vi "EIP IO Folder.vi"(8 "error in (no error)":errorcluster, 11 "Node Ptr":T1 format="%.0x") -> (0 "error out":errorcluster)   [LabVIEW 2011, in "Ethernet IP Custom Device Custom Device.lvlib"]
uses:
  Ethernet IP Custom Device Custom Device.lvlib
  <vilib>/NI Veristand/Custom Device API/Custom Device Item Ref.ctl
  <vilib>/NI Veristand/Custom Device API/Custom Device Channel.ctl
  <vilib>/NI Veristand/Custom Device API/Custom Device Channel Type.ctl
  Ethernet IP Global Strings.vi
  <vilib>/NI Veristand/Custom Device API/Get Item Property (Boolean).vi
  Ethernet IP Global GUIDs.vi
  <vilib>/NI Veristand/Custom Device API/Custom Device API.lvlib
panel:
  in  "Add Channel":bool
  in  "Header":cluster{"Section Name":string}={"Section Name"="Custom Device Item Settings"}
  out "Description":string
  out "Name":string
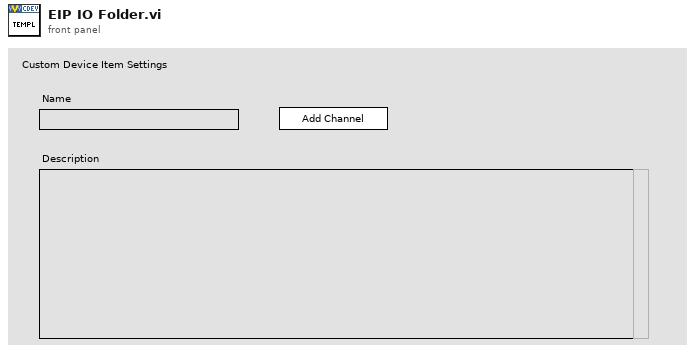
[diagram p1: front panel]
types:
  T1 = typedef "Custom Device API.lvlib/Custom Device Item Ref.ctl" = u64
  T2 = typedef "Custom Device API.lvlib/Custom Device Item Info.ctl" = cluster{"Name":string, "Is Channel":bool, "GUID":string}
  T3 = typedef "Custom Device API.lvlib/Custom Device Channel.ctl" = cluster{"Type":T4, "Units":string, "Default Value":dbl, "Faultable":bool, "Scalable":bool}
  T4 = typedef "Custom Device API.lvlib/Custom Device Channel Type.ctl" = enum16{"Input", "Output"}
  T5 = typedef "Custom Device API.lvlib/Custom Device Commands.ctl" = enum16{"Default", "Item renamed", "Shutdown", "Dynamic button pressed"}
  T6 = typedef "Ethernet IP Custom Device Custom Device.lvlib/L5K Data Types.ctl" = enum16{"SINT", "INT", "DINT", "REAL", "BOOL"}
  T7 = cluster{"Channel Name":string, "Tag Name":string, "Number of Elements":u16, "Data Type":T6}
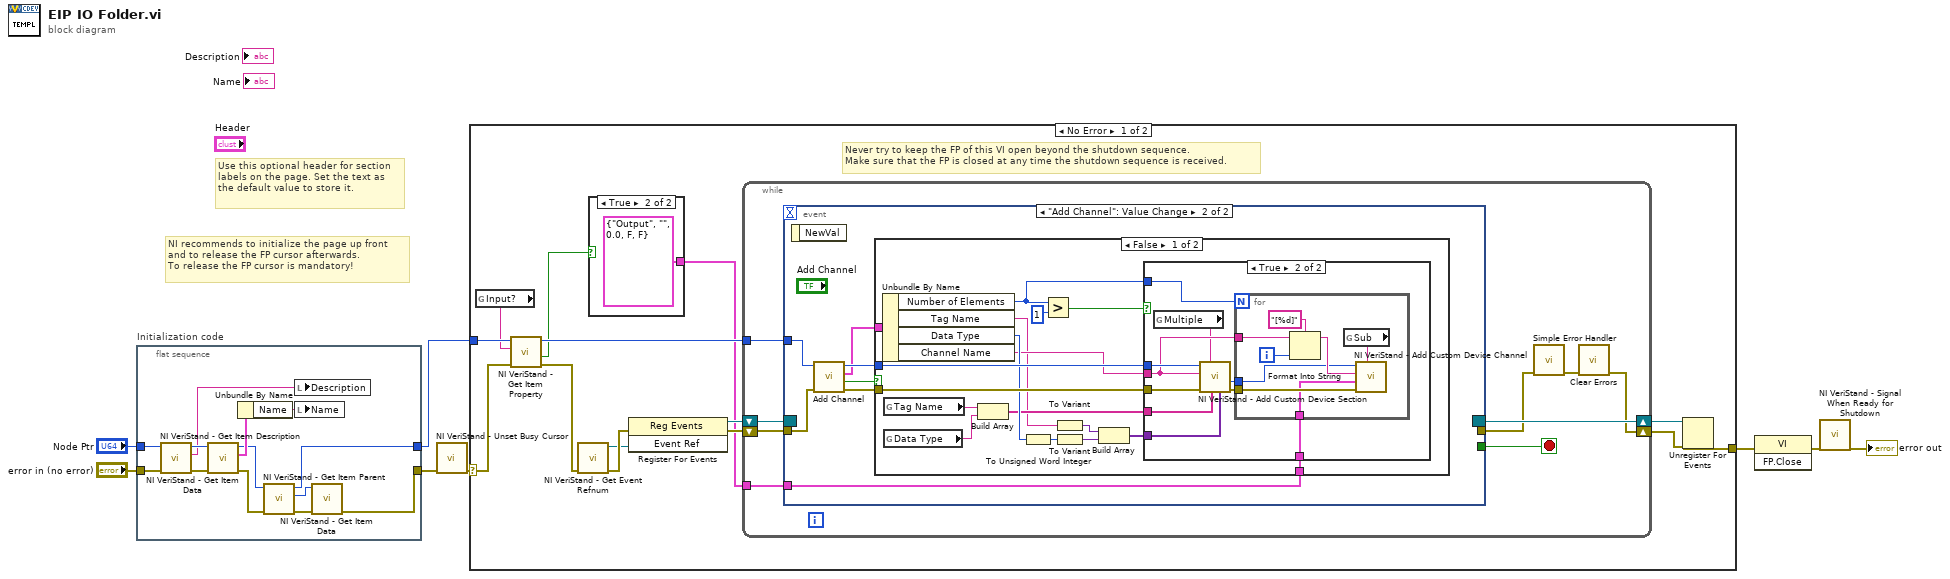
[diagram p0: block diagram]
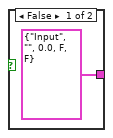
[diagram p2: hidden frame]
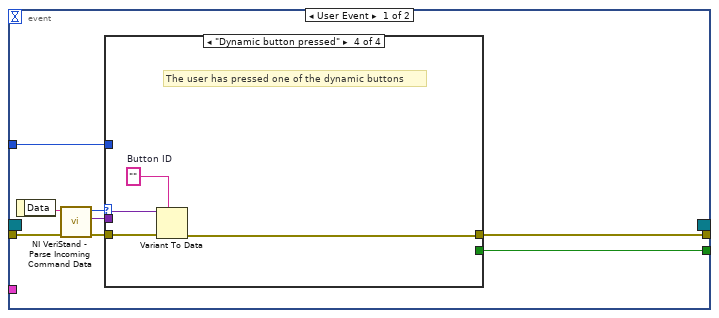
[diagram p3: hidden frame]
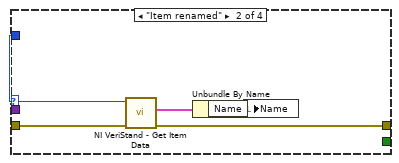
[diagram p5: hidden frame]
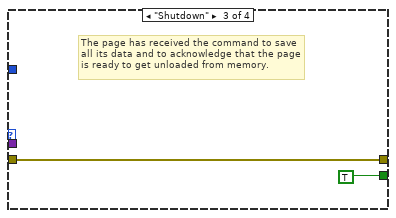
[diagram p6: hidden frame]
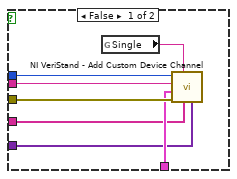
[diagram p7: hidden frame]
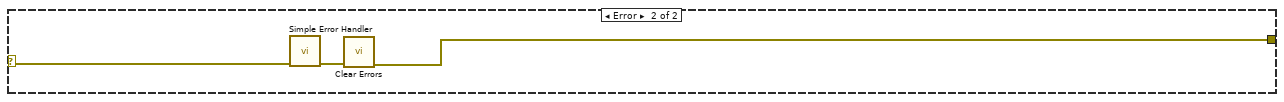
[diagram p9: hidden frame]
diagram:
  # "Use this optional header for section labels on the page. Set the text as the default value to store it."
  # "NI recommends to initialize the page up front\nand to release the FP cursor afterwards.\nTo release the FP cursor is mandatory!"
  n1 = flat-sequence "Initialization code" {
    tunnel: "error in (no error)" -> [w20]
    tunnel: "Node Ptr" -> [w19]
    tunnel: [w12] -> w2
    tunnel: [w10] -> w1
    frame #0 {
      n2 = call <vilib>:"NI VeriStand - Get Item Description.vi"("error in (no error)"=w20, "Item Ref in"=w19) -> ("error out"=w17:errorcluster, "Description"=w18:string, "Item Ref out"=w21:T1)  [unwired: 7 out]
      n3 = call <vilib>:"NI VeriStand - Get Item Data.vi"("error in (no error)"=w17, "Item Ref in"=w21) -> ("error out"=w14:errorcluster, "Item Info"=w16:T2, "Item Ref out"=w13:T1)  [unwired: 7 out]
      n4 = Unbundle By Name(w16) -> ("Name"=w15:string)
      n5 = call <vilib>:"NI VeriStand - Get Item Parent.vi"("error in (no error)"=w14, "Item Ref in"=w13) -> ("error out"=w11:errorcluster, "Parent Ref"=w9:T1, "Item Ref out"=w12:T1)  [unwired: 6 in, 1 out]
      n6 = local write "Description"(w18) -> ()
      n7 = local write "Name"(w15) -> ()
      n8 = call <vilib>:"NI VeriStand - Get Item Data.vi"("error in (no error)"=w11, "Item Ref in"=w9) -> ("error out"=w10:errorcluster)  [unwired: 6 in, 3 out]
    }
  }
  n9 = call <vilib>:"NI VeriStand - Unset Busy Cursor.vi"("error in (no error)"=w1) -> ("error out"=w4:errorcluster)  [unwired: 10 out]
  n10 = case shown="No Error" w4 {
    selector: w4 -> [w26 w118]
    tunnel: [w32 w116] -> w8
    tunnel: w2 -> [w28 _]
    frame No Error {
      # "Never try to keep the FP of this VI open beyond the shutdown sequence.\nMake sure that the FP is closed at any time the shutdown sequence is received."
      n11 = global read "Ethernet IP Global Strings.vi" "Input?"() -> (w22:string)
      n12 = call-poly <vilib>:"NI VeriStand - Get Item Property.vi"("error in (no error)"=w26, "Property Name"=w22, "Item Ref in"=w28) -> ("error out"=w25:errorcluster, "Value"=w24:bool, "Item Ref out"=w27:T1)  [unwired: 5 in, 1 out]
      n13 = call <vilib>:"NI VeriStand - Get Event Refnum.vi"("error in (no error)"=w25) -> ("error out"=w35:errorcluster, "Event Ref"=w31:refnum<user-event>)  [unwired: 9 out]
      n14 = case shown="True" w24 {
        tunnel: [T3 {"Type"=enum."Input", "Units"="", "Default Value"=0.0, "Faultable"=FALSE, "Scalable"=FALSE} ("Channel") T3 {"Type"=enum."Output", "Units"="", "Default Value"=0.0, "Faultable"=FALSE, "Scalable"=FALSE} ("Channel")] -> w23
        frame False {
        }
        frame True {
        }
      }
      n15 = register-events(error in=w35, w31) -> (reference out=w29:refnum<event-registration>, error out=w30:errorcluster)  [unwired: 1 in]
      n16 = while {
        tunnel: w27 -> [w42]
        shift-right: [w39] -> w33
        shift-left: w30 -> [w45]
        shift-right: [w46] -> w34
        shift-left: w29 -> [w44]
        tunnel: w23 -> [w38]
        stop <- w43 stop-if-true
        n17 = event shown="[1] \"Add Channel\": Value Change" {
          selector: w44 -> [_ _]
          dyn-events: [_ _] -> w46
          timeout: _ -> [_ _]
          tunnel: w45 -> [w54 w72]
          tunnel: [w50 _] -> w43
          tunnel: [w49 _] -> w41
          tunnel: w42 -> [w48 w73]
          tunnel: w38 -> [_ w67]
          event User Event {
            n18 = event-data() -> ("Data"=w53:string)  [unwired: 1 out]
            n19 = call <vilib>:"NI VeriStand - Parse Incoming Command Data.vi"("error in (no error)"=w54, "Incoming data"=w53) -> ("error out"=w52:errorcluster, "Outgoing data"=w47:variant, "Action"=w51:T5)  [unwired: 7 out]
            n20 = case shown="\"Dynamic button pressed\"" w51 {
              tunnel: w52 -> [w55 w60 w61 w66]
              tunnel: [_ _ TRUE _] -> w50
              tunnel: [w55 w57 w61 w63] -> w49
              tunnel: w48 -> [_ w59 _ _]
              tunnel: w47 -> [_ _ _ w65]
              frame "Default", Default {
              }
              frame "Item renamed" {
                n21 = call <vilib>:"NI VeriStand - Get Item Data.vi"("error in (no error)"=w60, "Item Ref in"=w59) -> ("error out"=w57:errorcluster, "Item Info"=w58:T2)  [unwired: 8 out]
                n22 = Unbundle By Name(w58) -> ("Name"=w56:string)
                n23 = local write "Name"(w56) -> ()
              }
              frame "Shutdown" {
                # "The page has received the command to save all its data and to acknowledge that the page is ready to get unloaded from memory."
              }
              frame "Dynamic button pressed" {
                w64 = ""  # Button ID
                # "The user has pressed one of the dynamic buttons"
                n24 = Variant To Data(error in=w66, type=w64, Variant=w65) -> (error out=w63:errorcluster)  [unwired: 1 out]
              }
            }
          }
          event "Add Channel": Value Change {
            n25 = event-data() -> ()  [unwired: 2 out]
            n26 = call "Add Channel.vi"("error in (no error)"=w72, "Parent Ref in"=w73) -> ("error out"=w71:errorcluster, "Cancelled?"=w69:bool, "Channel Settings"=w68:T7, "Parent Ref out"=w70:T1)  [unwired: 6 in]
            n27 = case shown="False" w69 {
              tunnel: w71 -> [w87 _]
              tunnel: w70 -> [w88 _]
              tunnel: w68 -> [w84 _]
              tunnel: w67 -> [w85 _]
              frame False {
                n28 = Unbundle By Name(w84) -> ("Number of Elements"=w86:u16, "Tag Name"=w76:string, "Data Type"=w82:T6, "Channel Name"=w79:string)
                n29 = global read "Ethernet IP Global Strings.vi" "Tag Name"() -> (w75:string)
                n30 = global read "Ethernet IP Global Strings.vi" "Data Type"() -> (w74:string)
                n31 = Build Array(w75, w74) -> (w80:string[])
                n32 = To Unsigned Word Integer(number=w82) -> (unsigned 16bit integer=w78:u16)
                n33 = Greater?(x=w86, y=u16 1) -> (0:w89:bool)
                n34 = To Variant(anything=w76) -> (Variant=w77:variant)
                n35 = To Variant(anything=w78) -> (Variant=w83:variant)
                n36 = Build Array(w77, w83) -> (w81:variant[])
                n37 = case shown="True" w89 {
                  tunnel: w88 -> [w97 w104]
                  tunnel: w87 -> [w96 w105]
                  tunnel: w86 -> [_ w101]
                  tunnel: w85 -> [w95 w99]
                  tunnel: w79 -> [w94 w100]
                  tunnel: w81 -> [w92 w107]
                  tunnel: w80 -> [w93 w106]
                  frame False {
                    n38 = global read "Ethernet IP Global GUIDs.vi" "Single"() -> (w91:string)
                    n39 = call <vilib>:"NI VeriStand - Add Custom Device Channel.vi"("Property Values"=w92, "Property names"=w93, "GUID (Default Channel)"=w91, "error in (no error)"=w96, "Channel"=w95, "Channel Name"=w94, "Parent Ref in"=w97) -> ()  [unwired: 1 in, 4 out]
                  }
                  frame True {
                    n40 = global read "Ethernet IP Global GUIDs.vi" "Multiple"() -> (w98:string)
                    n41 = call <vilib>:"NI VeriStand - Add Custom Device Section.vi"("Property Values"=w107, "Property names"=w106, "GUID (Default Section)"=w98, "error in (no error)"=w105, "Section Name"=w100, "Parent Ref in"=w104) -> ("error out"=w102:errorcluster, "Section Ptr"=w103:T1)  [unwired: 2 in, 2 out]
                    n42 = for {
                      N: w101 -> [_]
                      tunnel: w103 -> [w110]
                      tunnel: w102 -> [w115]
                      tunnel: w100 -> [w113]
                      tunnel: w99 -> [w109]
                      i -> [w114]
                      n43 = Format Into String(format string="[%d]", initial string=w113, w114) -> (resulting string=w111:string)  [unwired: 1 in, 1 out]
                      n44 = global read "Ethernet IP Global GUIDs.vi" "Sub"() -> (w108:string)
                      n45 = call <vilib>:"NI VeriStand - Add Custom Device Channel.vi"("GUID (Default Channel)"=w108, "error in (no error)"=w115, "Channel"=w109, "Channel Name"=w111, "Parent Ref in"=w110) -> ()  [unwired: 3 in, 4 out]
                    }
                  }
                }
              }
              frame True {
              }
            }
          }
        }
        n46 = call <vilib>:"Simple Error Handler.vi"("error in (no error)"=w41) -> ("error out"=w40:errorcluster)  [unwired: 1 in, 7 out]
        n47 = call <vilib>:"Clear Errors.vi"("error in (no error)"=w40) -> ("error out"=w39:errorcluster)  [unwired: 6 out]
      }
      n48 = Unregister For Events(event registration refnum=w34, error in=w33) -> (error out=w32:errorcluster)
    }
    frame Error {
      n49 = call <vilib>:"Simple Error Handler.vi"("error in (no error)"=w118) -> ("error out"=w117:errorcluster)  [unwired: 1 in, 7 out]
      n50 = call <vilib>:"Clear Errors.vi"("error in (no error)"=w117) -> ("error out"=w116:errorcluster)  [unwired: 6 out]
    }
  }
  n51 = invoke class="VI" method="FP.Close"(error in=w8) -> (error out=w7:errorcluster)  [unwired: 2 in, 2 out]
  n52 = call <vilib>:"NI VeriStand - Signal When Ready for Shutdown.vi"("error in (no error)"=w7) -> ("error out"=→"error out":errorcluster)  [unwired: 10 out]
